vi "UpdateTimerToCaller.vi"(8 "error in (no error)":errorcluster, 11 "Timer_Event in":refnum<class "Timer_Event.lvclass">) -> (0 "error out":errorcluster, 3 "Timer_Event out":refnum<class "Timer_Event.lvclass">)   [LabVIEW 2020, in "Timer_Event.lvlib" / "Timer_Event.lvclass"]
uses:
  Timer_Event.lvclass
  C:/Program Files (x86)/National Instruments/LabVIEW 2020/vi.lib/ActorFramework/Actor/Actor.lvclass
  <vilib>/ActorFramework/Actor/Actor.lvclass/Actor.ctl
  Timer_Event.lvclass/Timer_Event.ctl
  Timer_Event Messages/UpdateTimeToParent Msg/UpdateTimeToParent Msg.lvclass/UpdateTimeToParent Msg.ctl
  <vilib>/ActorFramework/Message Enqueuer/Message Enqueuer.lvclass/Message Enqueuer.ctl
  <vilib>/ActorFramework/Message Enqueuer/Enqueue.vi
  Timer_Event Messages/UpdateTimeToParent Msg/UpdateTimeToParent Msg.lvclass
  C:/Program Files (x86)/National Instruments/LabVIEW 2020/vi.lib/ActorFramework/Message/Message.lvclass
  <vilib>/ActorFramework/Message Priority Queue/Priority Enqueue.vi
  <vilib>/ActorFramework/Actor/Actor.lvclass
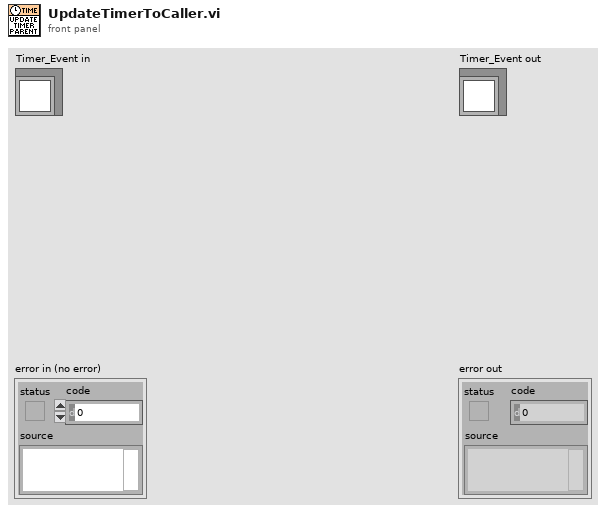
[diagram p1: front panel]
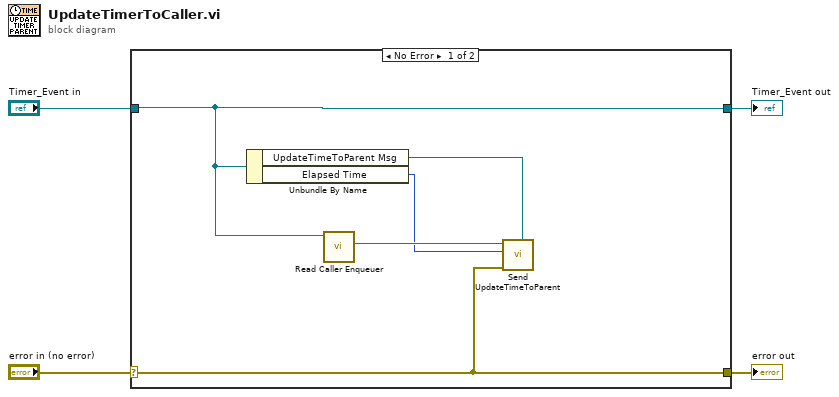
[diagram p0: block diagram]
diagram:
  n1 = case shown="No Error" "error in (no error)" {
    selector: "error in (no error)" -> [w5 w11]
    tunnel: [w5 w11] -> w3
    tunnel: [w9 w10] -> w1
    tunnel: "Timer_Event in" -> [w9 w10]
    frame No Error {
      n2 = Unbundle By Name(w9) -> ("UpdateTimeToParent Msg"=w7:refnum<class "UpdateTimeToParent Msg.lvclass">, "Elapsed Time"=w6:i32)
      n3 = call <vilib>:"Read Caller Enqueuer.vi"("Actor"=w9) -> ("Caller Enqueuer"=w8:refnum<class "Message Enqueuer.lvclass">)  [unwired: 10 in]
      n4 = call "Send UpdateTimeToParent.vi"("Message Type"=w7, "error in (no error)"=w5, "ElapsedTime"=w6, "Message Enqueuer"=w8) -> ()  [unwired: 6 in, 2 out]
    }
    frame Error {
    }
  }
  "error out" <- w3
  "Timer_Event out" <- w1
